vi "Read Analogue.vi"(8 "error in (no error)":errorcluster, 11 "PS in":refnum<class "APS7050.lvclass">) -> (0 "error out":errorcluster, 2 "Measurements":dbl, 3 "PS out":refnum<class "APS7050.lvclass">)   [LabVIEW 2019, in "Concrete.lvlib" / "APS7050.lvclass"]
uses:
  APS7050.lvclass
  APS7050.lvclass/APS7050.ctl
  Harware Abstraction/Analog out/Analog out.lvclass
  <instrlib>/APS-7000 Series/APS-7000 Series.lvlib
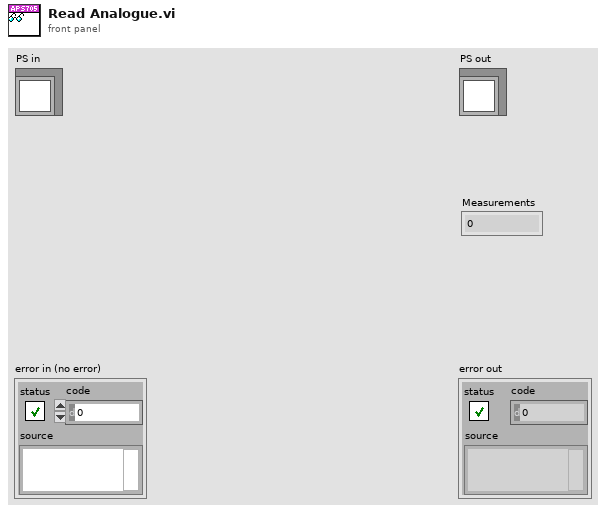
[diagram p1: front panel]
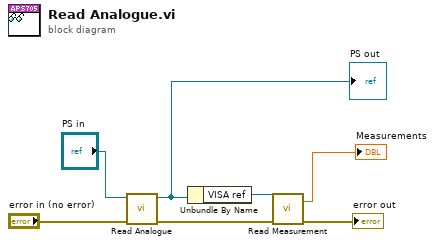
[diagram p0: block diagram]
diagram:
  n1 = call-parent "Read Analogue.vi"("error in (no error)"="error in (no error)", "Analog out in"="PS in") -> ("error out"=w5:errorcluster, "Analog out out"=w3:refnum<class "APS7050.lvclass">)  [unwired: 7 in, 1 out]
  "PS out" <- w3
  n2 = Unbundle By Name(w3) -> ("VISA ref"=w2:refnum<visa-resource-name>)
  n3 = call <instrlib>:"Read Measurement.vi"("VISA in"=w2, "error in"=w5) -> ("Power? (W)"=→"Measurements":dbl, "error out"=→"error out":errorcluster)  [unwired: 3 in, 9 out]
